vi "读取固件状态.vi"(8 "错误输入":errorcluster, 11 "MB session in":refnum<class "MB_Master.lvclass">) -> (0 "error out":errorcluster, 2 "结果字符串":string, 3 "MB session out":refnum<class "MB_Master.lvclass">)   [LabVIEW 2016, in "斯坦道CODMn新电路板.lvlib"]
uses:
  <vilib>/Plasmionique/MB Master/MB_Master/MB_Master.lvclass
  <vilib>/Plasmionique/MB Master/MB_Master_Serial/MB_Master_Serial.lvclass
  C:/Program Files (x86)/National Instruments/LabVIEW 2016/vi.lib/Plasmionique/MB Master/MB_Master/MB_Master.lvclass
  <vilib>/Plasmionique/MB Master/MB Master.lvlib
panel:
  in  "VISA Resource":refnum<visa-resource-name>
  in  "引用选择":enum16{"MB引用", "自建引用"}(ring)
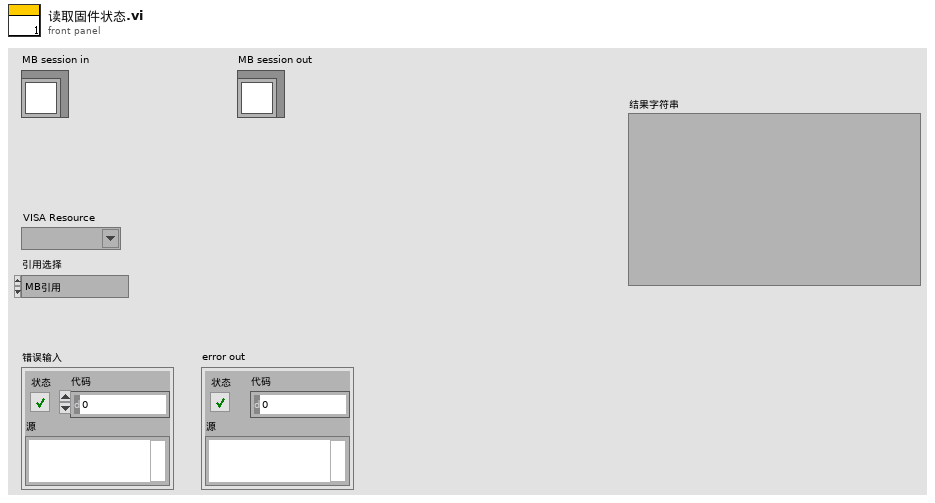
[diagram p1: front panel]
types:
  T1 = cluster{"baud rate (bps)":u32, "stop bits":u16, "parity":u16, "flow control":u16, "timeout":u32, "retries":i32}
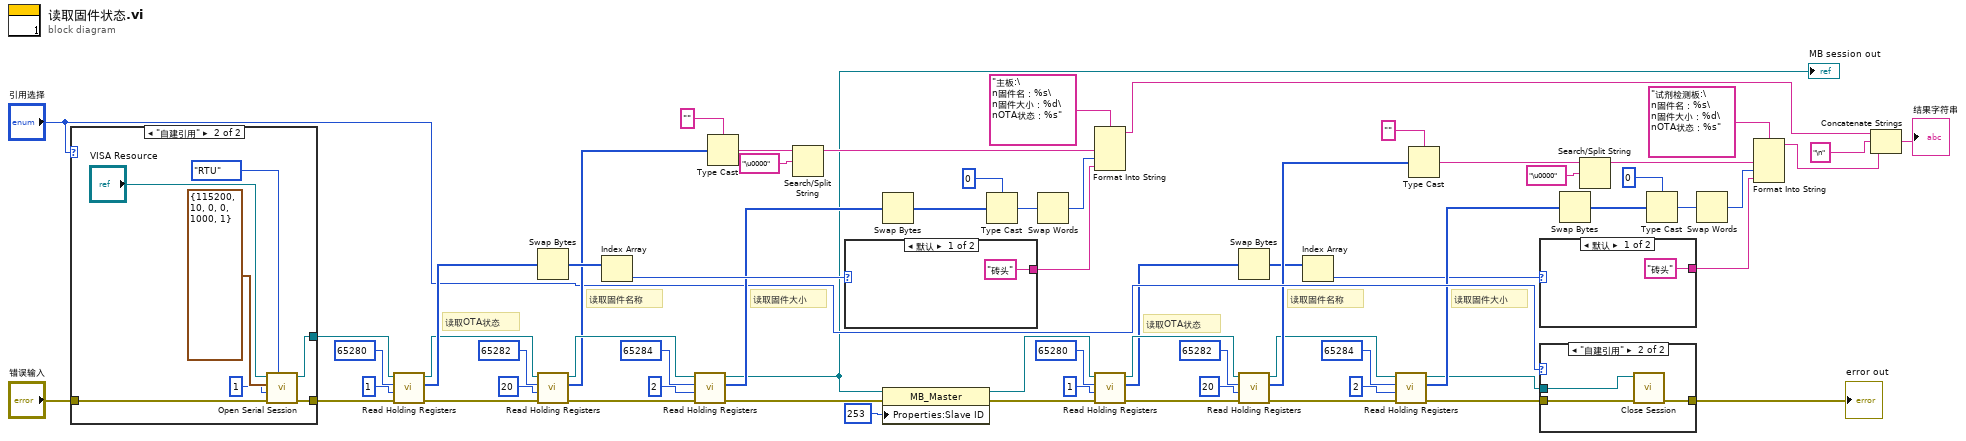
[diagram p0: block diagram]
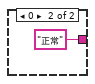
[diagram p2: hidden frame]
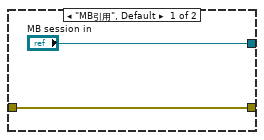
[diagram p4: hidden frame]
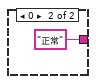
[diagram p5: hidden frame]
diagram:
  # "读取固件大小"
  # "读取固件名称"
  # "读取OTA状态"
  # "读取固件大小"
  # "读取固件名称"
  # "读取OTA状态"
  n1 = case shown="\"自建引用\"" "引用选择" {
    tunnel: ["MB session in" w74] -> w65
    tunnel: "错误输入" -> [w67 w73]
    tunnel: [w67 w72] -> w45
    frame "MB引用", Default {
    }
    frame "自建引用" {
      n2 = call <vilib>:"Open Serial Session.vi"("Mode (RTU)"=enum16{"RTU", "ASCII"}."RTU", "Error in"=w73, "Slave ID"=u8 1, "Serial Config"=T1 {"baud rate (bps)"=115200, "stop bits"=10, "parity"=0, "flow control"=0, "timeout"=1000, "retries"=1}, "VISA Resource"="VISA Resource") -> ("Error out"=w72:errorcluster, "MB_Serial session"=w74:refnum<class "MB_Master_Serial.lvclass">)  [unwired: 5 in]
    }
  }
  n3 = call <vilib>:"Read Holding Registers.vi"("error in (no error)"=w45, "quantity"=u16 1, "starting address"=u16 65280, "MB session in"=w65) -> ("error out"=w53:errorcluster, "Registers"=w62:u16[], "MB session out"=w58:refnum<class "MB_Master.lvclass">)  [unwired: 5 in]
  n4 = Swap Bytes(anything=w62) -> (byte swapped=w60:u16[])
  n5 = call <vilib>:"Read Holding Registers.vi"("error in (no error)"=w53, "quantity"=u16 20, "starting address"=u16 65282, "MB session in"=w58) -> ("error out"=w52:errorcluster, "Registers"=w39:u16[], "MB session out"=w56:refnum<class "MB_Master.lvclass">)  [unwired: 5 in]
  n6 = Index Array(array=w60) -> (element=w61:u16)  [unwired: 1 in]
  n7 = call <vilib>:"Read Holding Registers.vi"("error in (no error)"=w52, "quantity"=u16 2, "starting address"=u16 65284, "MB session in"=w56) -> ("error out"=w3:errorcluster, "Registers"=w51:u16[], "MB session out"=w7:refnum<class "MB_Master.lvclass">)  [unwired: 5 in]
  "MB session out" <- w7
  n8 = Type Cast(type="", x=w39) -> (*(type *) &x=w40:string)
  n9 = Search/Split String(string=w40, search string/char (-)="\u0000" ("搜索字符串")) -> (substring before match=w42:string)  [unwired: 1 in, 2 out]
  n10 = case shown="默认" w61 {
    tunnel: ["砖头" "正常"] -> w59
    frame Default {
    }
    frame 0 {
    }
  }
  n11 = Swap Bytes(anything=w51) -> (byte swapped=w50:u16[])
  n12 = property class="MB_Master"(reference=w7, error in=w3, "Properties:Slave ID"=u8 253 ("Slave ID")) -> (reference out=w5:refnum<class "MB_Master.lvclass">, error out=w4:errorcluster)
  n13 = Type Cast(type=u32 0, x=w50) -> (*(type *) &x=w48:u32)
  n14 = Swap Words(1:w48) -> (0:w47:u32)
  n15 = Format Into String(format string="主板:\n固件名：%s\n固件大小：%d\nOTA状态：%s" ("格式字符串"), w42, w47, w59) -> (resulting string=w35:string)  [unwired: 2 in, 1 out]
  n16 = call <vilib>:"Read Holding Registers.vi"("error in (no error)"=w4, "quantity"=u16 1, "starting address"=u16 65280, "MB session in"=w5) -> ("error out"=w23:errorcluster, "Registers"=w15:u16[], "MB session out"=w18:refnum<class "MB_Master.lvclass">)  [unwired: 5 in]
  n17 = Swap Bytes(anything=w15) -> (byte swapped=w17:u16[])
  n18 = call <vilib>:"Read Holding Registers.vi"("error in (no error)"=w23, "quantity"=u16 20, "starting address"=u16 65282, "MB session in"=w18) -> ("error out"=w24:errorcluster, "Registers"=w33:u16[], "MB session out"=w20:refnum<class "MB_Master.lvclass">)  [unwired: 5 in]
  n19 = Index Array(array=w17) -> (element=w16:u16)  [unwired: 1 in]
  n20 = call <vilib>:"Read Holding Registers.vi"("error in (no error)"=w24, "quantity"=u16 2, "starting address"=u16 65284, "MB session in"=w20) -> ("error out"=w8:errorcluster, "Registers"=w25:u16[], "MB session out"=w9:refnum<class "MB_Master.lvclass">)  [unwired: 5 in]
  n21 = Type Cast(type="", x=w33) -> (*(type *) &x=w32:string)
  n22 = case shown="默认" w16 {
    tunnel: ["砖头" "正常"] -> w12
    frame Default {
    }
    frame 0 {
    }
  }
  n23 = case shown="\"自建引用\"" "引用选择" {
    tunnel: w9 -> [_ w83]
    tunnel: w8 -> [w80 w82]
    tunnel: [w80 w81] -> w34
    frame "MB引用", Default {
    }
    frame "自建引用" {
      n24 = call-dynamic "Close Session.vi"("error in (no error)"=w82, "MB session in"=w83) -> ("error out"=w81:errorcluster)  [unwired: 9 in]
    }
  }
  "error out" <- w34
  n25 = Swap Bytes(anything=w25) -> (byte swapped=w26:u16[])
  n26 = Search/Split String(string=w32, search string/char (-)="\u0000" ("搜索字符串")) -> (substring before match=w10:string)  [unwired: 1 in, 2 out]
  n27 = Type Cast(type=u32 0, x=w26) -> (*(type *) &x=w28:u32)
  n28 = Swap Words(1:w28) -> (0:w11:u32)
  n29 = Format Into String(format string="试剂检测板:\n固件名：%s\n固件大小：%d\nOTA状态：%s" ("格式字符串"), w10, w11, w12) -> (resulting string=w1:string)  [unwired: 2 in, 1 out]
  n30 = Concatenate Strings(w35, "\n", w1) -> (→"结果字符串":string)
